vi "Swerve Controller Interactive Check.vi"(8 "Interactive Command in":T1 {"CHASSIS"."vOmega" format="%10.3f"; "CHASSIS"."vY" format="%10.3f"; "CHASSIS"."vX" format="%10.3f"}, 9 "Default Command":T1 {"CHASSIS"."vOmega" format="%10.3f"; "CHASSIS"."vY" format="%10.3f"; "CHASSIS"."vX" format="%10.3f"}, 11 "Buttons":cluster{"Execute Cmd":bool, "Abort Cmd":bool}) -> (1 "Interactive Command out":T1 {"CHASSIS"."vOmega" format="%10.3f"; "CHASSIS"."vY" format="%10.3f"; "CHASSIS"."vX" format="%10.3f"}, 2 "Trace String":string, 3 "Schedule":bool)   [LabVIEW 2023]
doc: "Check the Execute and Abort buttons and choose the data and trace string."
uses:
  Swerve Setpoints.ctl
  Swerve Operations.ctl
  <vilib>/Rock Robotics/WPI/ThirdParty/JAS_Junk/TrajLib/TypeDef/CHASSIS_SPEEDS.ctl
  <vilib>/Rock Robotics/WPI/ThirdParty/JAS_Junk/TrajLib/Trajectory_Library.lvlib
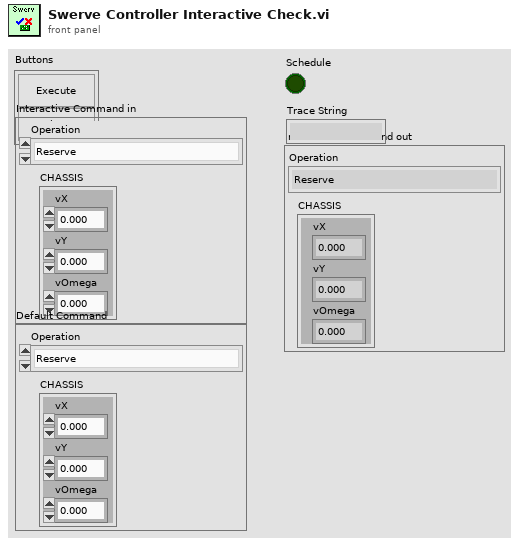
[diagram p1: front panel]
types:
  T1 = typedef "Swerve Setpoints.ctl" = cluster{"Operation":T2, "CHASSIS":T3}
  T2 = typedef "Swerve Operations.ctl" = enum16{"Reserve", "Read Current", "Immediate", "Joystick Drive"}
  T3 = typedef "Trajectory_Library.lvlib/CHASSIS_SPEEDS.ctl" = cluster{"vX":dbl, "vY":dbl, "vOmega":dbl}
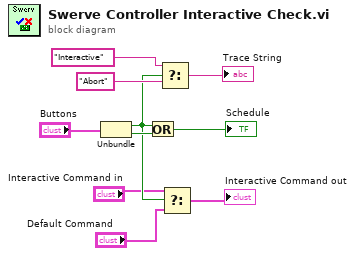
[diagram p0: block diagram]
diagram:
  n1 = Unbundle("Buttons") -> ("Execute Cmd"=w6:bool, "Abort Cmd"=w7:bool)
  n2 = Or(x=w6, y=w7) -> (x .or. y?=→"Schedule":bool)
  n3 = Select(t="Interactive", s=w6, f="Abort") -> (s? t:f=→"Trace String":string)
  n4 = Select(t="Interactive Command in", s=w6, f="Default Command") -> (s? t:f=→"Interactive Command out":T1)
